vi "Get Temperatures.vi"(7 "1-Wire DIO Pin":refnum<k21>, 8 "error in (no error)":errorcluster, 10 "ROM Array":u64[](array[numeric])=[0, 0, 0, 0, 0, 0, 0, 0]) -> (0 "error out":errorcluster, 2 "Temperature Array":u16[](array[numeric]))   [LabVIEW 2014, in "Maxim 1-Wire.lvlib"]
doc: "Attempts a RESET -> MATCH ROM -> CONVERT T -> RESET -> MATCH ROM -> READ SCRATCHPAD cycle for every ROM in ROM Array and returns the first word of the scratchpad (which contains the two temperature bytes)."
uses:
  Maxim 1-Wire.lvlib
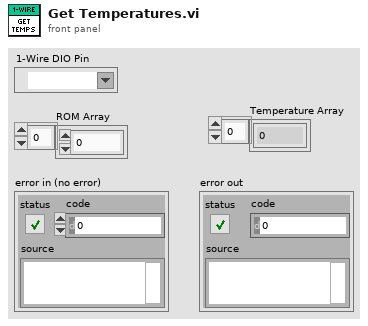
[diagram p1: front panel]
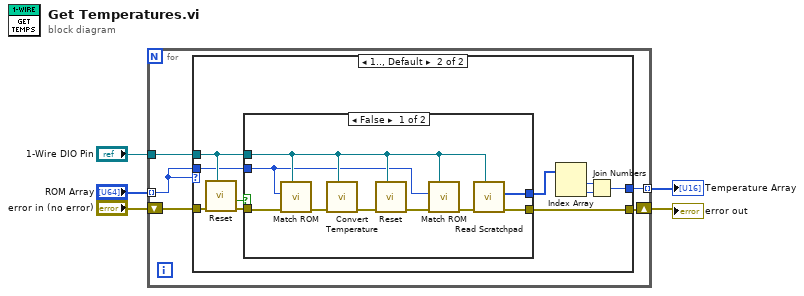
[diagram p0: block diagram]
diagram:
  n1 = for {
    shift-right: [w8] -> w1
    shift-left: "error in (no error)" -> [w10]
    tunnel: "ROM Array" -> [w6] mode=indexing
    tunnel: "1-Wire DIO Pin" -> [w9]
    tunnel: [w7] -> w2 mode=indexing
    n2 = case shown="1.., Default" w6 {
      tunnel: w10 -> [w11 w21]
      tunnel: w9 -> [_ w18]
      tunnel: [w11 w17] -> w8
      tunnel: w6 -> [_ w16]
      tunnel: [_ w13] -> w7
      frame 0 {
      }
      frame 1.., Default {
        n3 = call "Reset.vi"("1-Wire DIO Pin"=w18, "error in"=w21) -> ("error out"=w19:errorcluster, "0 = Device Present / 1=no"=w20:bool)  [unwired: 8 in]
        n4 = case shown="False" w20 {
          tunnel: w18 -> [w24 _]
          tunnel: w19 -> [w29 w31]
          tunnel: [w30 w31] -> w17
          tunnel: w16 -> [w23 _]
          tunnel: [w28 _] -> w12
          frame False {
            n5 = call "Match ROM.vi"("1-Wire DIO Pin"=w24, "error in (no error)"=w29, "ROM Code"=w23) -> ("error out"=w27:errorcluster)  [unwired: 8 in]
            n6 = call "Convert Temperature.vi"("1-Wire DIO Pin"=w24, "error in (no error)"=w27) -> ("error out"=w26:errorcluster)  [unwired: 8 in, 1 out]
            n7 = call "Reset.vi"("1-Wire DIO Pin"=w24, "error in"=w26) -> ("error out"=w25:errorcluster)  [unwired: 8 in, 1 out]
            n8 = call "Match ROM.vi"("1-Wire DIO Pin"=w24, "error in (no error)"=w25, "ROM Code"=w23) -> ("error out"=w22:errorcluster)  [unwired: 8 in]
            n9 = call "Read Scratchpad.vi"("1-Wire DIO Pin"=w24, "error in (no error)"=w22) -> ("error out"=w30:errorcluster, "Scratchpad Data"=w28:u8[])  [unwired: 7 in]
          }
          frame True {
          }
        }
        n10 = Index Array(array=w12) -> (element #1=w14:u8, element #2=w15:u8)  [unwired: 2 in]
        n11 = Join Numbers(hi=w14, lo=w15) -> ((hi.lo)=w13:u16)
      }
    }
  }
  "Temperature Array" <- w2
  "error out" <- w1
